vi "Format Logging Properties.vi"(11 "Logging properties":T1) -> (3 "Logging string":string)   [LabVIEW 2015, in "NI_Azure_Queue.lvlib"]
uses:
  NI_Azure_Queue.lvlib
  Logging.ctl
  Retention Policy.ctl
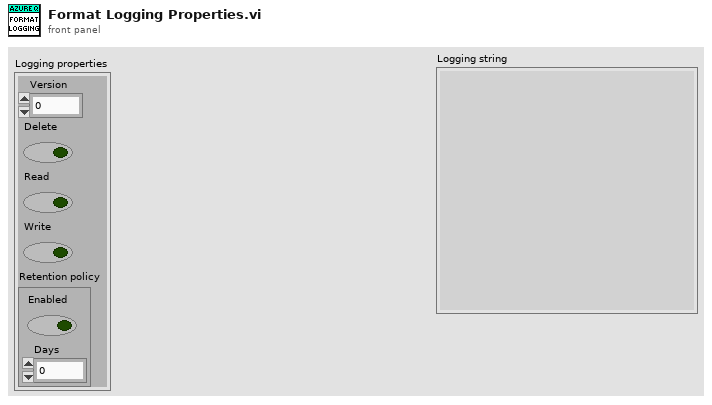
[diagram p1: front panel]
types:
  T1 = typedef "NI_Azure_Queue.lvlib/Logging.ctl" = cluster{"Version":dbl, "Delete":bool, "Read":bool, "Write":bool, "Retention policy":T2}
  T2 = typedef "NI_Azure_Queue.lvlib/Retention Policy.ctl" = cluster{"Enabled":bool, "Days":u32}
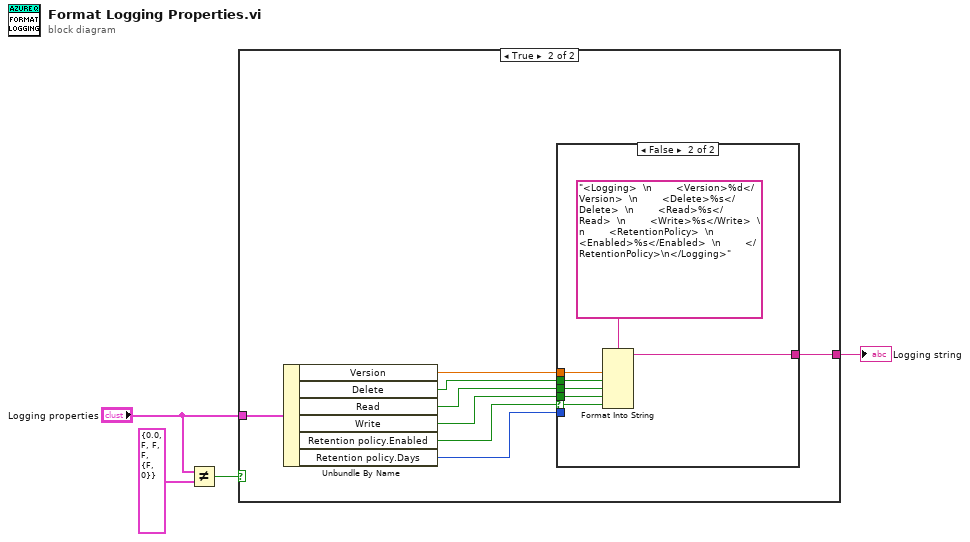
[diagram p0: block diagram]
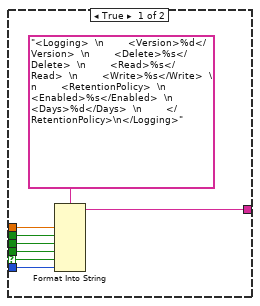
[diagram p3: hidden frame]
diagram:
  n1 = Not Equal?(x="Logging properties", y=T1 {"Version"=0.0, "Delete"=FALSE, "Read"=FALSE, "Write"=FALSE, "Retention policy"={"Enabled"=FALSE, "Days"=0}} ("Logging")) -> (x != y?=w3:bool)
  n2 = case shown="True" w3 {
    tunnel: "Logging properties" -> [_ w12]
    tunnel: [_ w5] -> w1
    frame False {
    }
    frame True {
      n3 = Unbundle By Name(w12) -> ("Version"=w11:dbl, "Delete"=w10:bool, "Read"=w9:bool, "Write"=w8:bool, "Retention policy.Enabled"=w7:bool, "Retention policy.Days"=w6:u32)
      n4 = case shown="False" w7 {
        selector: w7 -> [w16 w23]
        tunnel: w11 -> [w20 w27]
        tunnel: w10 -> [w19 w26]
        tunnel: w9 -> [w18 w25]
        tunnel: w8 -> [w17 w24]
        tunnel: w6 -> [w15 _]
        tunnel: [w14 w22] -> w5
        frame True {
          n5 = Format Into String(format string="<Logging>  \n        <Version>%d</Version>  \n        <Delete>%s</Delete>  \n        <Read>%s</Read>  \n        <Write>%s</Write>  \n        <RetentionPolicy>  \n            <Enabled>%s</Enabled>  \n            <Days>%d</Days>  \n        </RetentionPolicy>\n</Logging>", w20, w19, w18, w17, w16, w15) -> (resulting string=w14:string)  [unwired: 2 in, 1 out]
        }
        frame False {
          n6 = Format Into String(format string="<Logging>  \n        <Version>%d</Version>  \n        <Delete>%s</Delete>  \n        <Read>%s</Read>  \n        <Write>%s</Write>  \n        <RetentionPolicy>  \n            <Enabled>%s</Enabled>  \n        </RetentionPolicy>\n</Logging>", w27, w26, w25, w24, w23) -> (resulting string=w22:string)  [unwired: 2 in, 1 out]
        }
      }
    }
  }
  "Logging string" <- w1
